vi "IO_PWM.vi"() -> (8 "PWM Ref":bool)   [LabVIEW 2024]
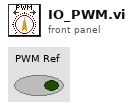
[diagram p1: front panel]
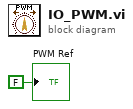
[diagram p0: block diagram]
diagram:
  "PWM Ref" <- FALSE ("DAQ Ref")
